vi "CryoServer Wait for Command Complete.vi"(8 "error in (no error)":errorcluster, 9 "Expect Response":string="CommandSucceeded", 10 "command string":string, 11 "connection ID":refnum<k5>) -> (0 "error out":errorcluster, 2 "Response":string, 3 "connection ID out":refnum<k5>)   [LabVIEW 2021, in "CryoServer.lvclass"]
uses:
  CryoServer.lvclass
  <vilib>/JDP Science/JSONtext/Next JSON Value.vi
  <vilib>/JDP Science/JSONtext/String Subset.vi
  <vilib>/JDP Science/JSONtext/Parsing/Advance past next JSON Value (inlined COPY).vi
  <vilib>/JDP Science/JSONtext/Parsing/Advance past whitespace.vi
  <vilib>/JDP Science/JSONtext/Parsing/Advance past String.vi
  <vilib>/JDP Science/JSONtext/Parsing/Advance past Number.vi
  <vilib>/JDP Science/JSONtext/Parsing/Advance past Line Ending.vi
  <vilib>/JDP Science/JSONtext/Parsing/Parse Full Path or Item Name.vi
  <vilib>/JDP Science/JSONtext/Parsing/Advance past Array.vi
  <vilib>/JDP Science/JSONtext/Parsing/Advance past Object.vi
  <vilib>/JDP Science/JSONtext/support/Error Cluster From Code.vi
  <vilib>/JDP Science/JSONtext/Offset/Find Item Locations by Path.vi
  <vilib>/JDP Science/JSONtext/JSONtext.lvlib
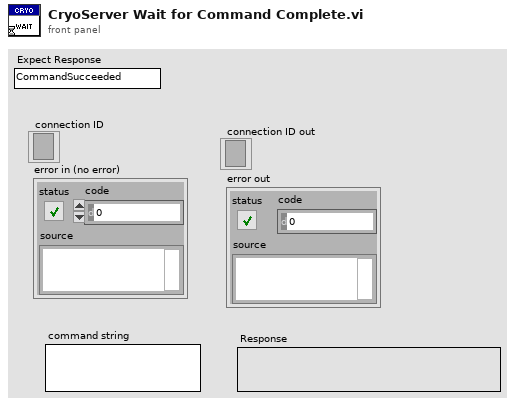
[diagram p1: front panel]
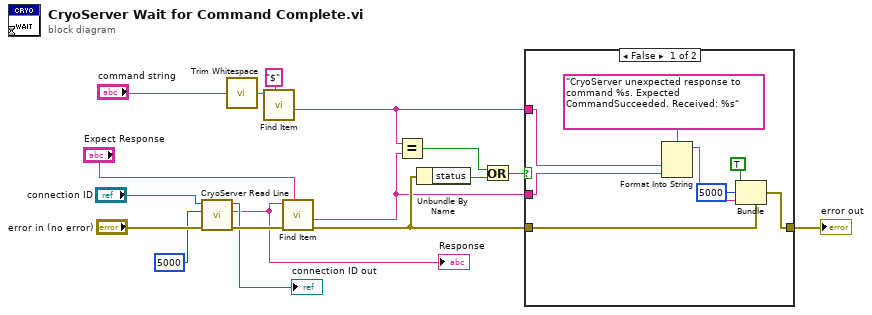
[diagram p0: block diagram]
diagram:
  n1 = call "CryoServer Read Line.vi"("error in (no error)"="error in (no error)", "timeout ms (5000)"=5000, "connection ID"="connection ID") -> ("error out"=w11:errorcluster, "data out"=w1:string, "connection ID out"=→"connection ID out":refnum<k5>)  [unwired: 6 in]
  "Response" <- w1
  n2 = call <vilib>:"Trim Whitespace.vi"("string"="command string") -> ("trimmed string"=w13:string)  [unwired: 1 in]
  n3 = call <vilib>:"Find Item.vi"("$Path or Item Name"="$", "JSON"=w13) -> ("<JSON>"=w4:string)  [unwired: 6 in, 3 out]
  n4 = call <vilib>:"Find Item.vi"("$Path or Item Name"="Expect Response", "error in (no error)"=w11, "JSON"=w1) -> ("error out"=w6:errorcluster, "<JSON>"=w3:string)  [unwired: 5 in, 2 out]
  n5 = Equal?(x=w4, y=w3) -> (x = y?=w8:bool)
  n6 = Unbundle By Name(w6) -> ("status"=w9:bool)
  n7 = Or(x=w8, y=w9) -> (x .or. y?=w7:bool)
  n8 = case shown="False" w7 {
    tunnel: w6 -> [w22 w26]
    tunnel: [w18 w26] -> w5
    tunnel: w4 -> [w24 _]
    tunnel: w3 -> [w23 _]
    frame False {
      n9 = Format Into String(format string="CryoServer unexpected response to command %s. Expected CommandSucceeded. Received: %s", w24, w23) -> (resulting string=w20:string)  [unwired: 2 in, 1 out]
      n10 = Bundle(cluster=w22, "status"=TRUE, "code"=5000, "source"=w20) -> (w18:errorcluster)
    }
    frame True {
    }
  }
  "error out" <- w5
